vi "Drivetrain.vi"(10 "Duration":i64, 11 "rt fifo":refnum<k33>) -> ()   [LabVIEW 2014]
uses:
  Drive Metrics.ctl
  Drive States.ctl
panel:
  in  "Drive Metrics":T1
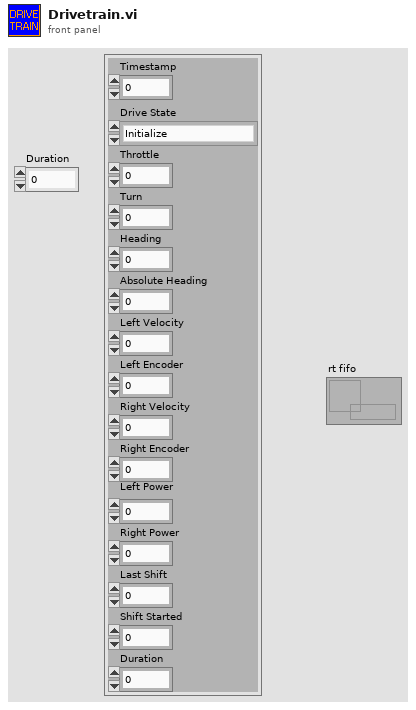
[diagram p1: front panel]
types:
  T1 = typedef "Drive Metrics.ctl" = cluster{"Timestamp":u32, "Drive State":T2, "Throttle":dbl, "Turn":dbl, "Heading":dbl, "Absolute Heading":dbl, "Left Velocity":dbl, "Left Encoder":dbl, "Right Velocity":dbl, "Right Encoder":dbl, "Left Power":dbl, "Right Power":dbl, "Last Shift":u32, "Shift Started":u32, "Duration":i64}
  T2 = typedef "Drive States.ctl" = enum16{"Initialize", "Low Gear", "Up Shift Begin", "Up Shifting", "Up Shift Delay", "High Gear", "Down Shift Begin", "Down Shifting", "Down Shift Delay"}
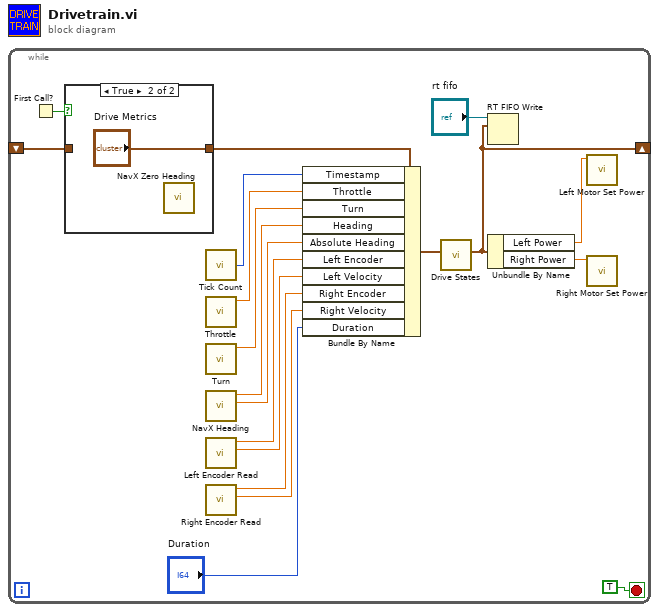
[diagram p0: block diagram]
diagram:
  n1 = while {
    shift-right: [w6] -> _
    shift-left: _ -> [w3]
    stop <- TRUE stop-if-true
    n2 = First Call?() -> (First Call?: T/F=w5:bool)
    n3 = case shown="True" w5 {
      tunnel: [w20 "Drive Metrics"] -> w4
      tunnel: w3 -> [w20 _]
      frame False {
      }
      frame True {
        n4 = call "NavX Zero Heading.vi"() -> ()  [unwired: 11 in, 1 out]
      }
    }
    n5 = call "Tick Count"() -> ("Tick Count(uSec)"=w1:u32)
    n6 = call "Throttle.vi"() -> ("throttle"=w18:dbl)  [unwired: 10 in, 1 out]
    n7 = call "Turn.vi"() -> ("turn"=w17:dbl)  [unwired: 10 in, 1 out]
    n8 = call "NavX Heading.vi"() -> ("Absolute Heading"=w9:dbl, "Heading"=w14:dbl)  [unwired: 9 in, 1 out]
    n9 = call "Left Encoder Read.vi"() -> ("Rate"=w8:dbl, "Distance"=w12:dbl)  [unwired: 8 in, 2 out]
    n10 = call "Right Encoder Read.vi"() -> ("Rate"=w7:dbl, "Distance"=w13:dbl)  [unwired: 8 in, 2 out]
    n11 = Bundle By Name(cluster=w4, "Timestamp"=w1, "Throttle"=w18, "Turn"=w17, "Heading"=w14, "Absolute Heading"=w9, "Left Encoder"=w12, "Left Velocity"=w8, "Right Encoder"=w13, "Right Velocity"=w7, "Duration"="Duration") -> (w10:T1)
    n12 = call "Drive States.vi"("Drive Metrics in"=w10) -> ("Drive Metrics out"=w6:T1)  [unwired: 10 in]
    n13 = RT FIFO Write(0:"rt fifo", 1:w6) -> ()  [unwired: 3 in, 4 out]
    n14 = Unbundle By Name(w6) -> ("Left Power"=w16:dbl, "Right Power"=w15:dbl)
    n15 = call "Left Motor Set Power.vi"("Output"=w16) -> ()  [unwired: 10 in, 1 out]
    n16 = call "Right Motor Set Power.vi"("Output"=w15) -> ()  [unwired: 10 in, 1 out]
  }
